vi "Re-Origin.vi"(1 "Transition":cluster{"X Delta":dbl, "Y Delta":dbl}, 2 "Coordinates":cluster{"X":dbl, "Y":dbl}[](array[cluster])) -> (0 "Normalized Coords":cluster{"X":dbl, "Y":dbl}[](array[cluster]))   [LabVIEW 2016]
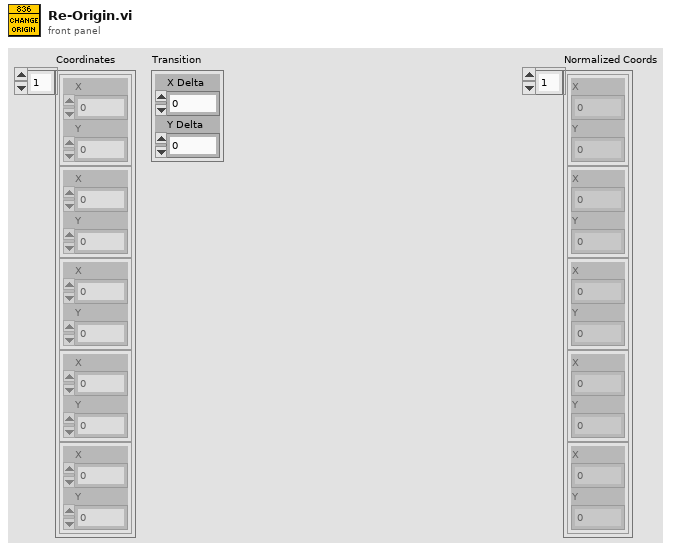
[diagram p1: front panel]
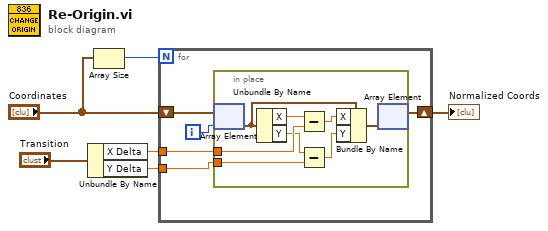
[diagram p0: block diagram]
diagram:
  n1 = Unbundle By Name("Transition") -> ("X Delta"=w3:dbl, "Y Delta"=w2:dbl)
  n2 = Array Size(array="Coordinates") -> (size(s)=w6:i32)
  n3 = for {
    N: w6 -> [_]
    tunnel: w3 -> [w9]
    tunnel: w2 -> [w8]
    shift-right: [w7] -> w1
    shift-left: "Coordinates" -> [w10]
    i -> [w11]
    n4 = in-place {
      in-place-border: w9 -> [w17]
      in-place-border: w8 -> [w15]
      n5 = in-place-array #1(w10, w11) -> (w18:cluster{"X":dbl, "Y":dbl})
      n6 = Unbundle By Name(w18) -> ("X"=w16:dbl, "Y"=w12:dbl)
      n7 = Subtract(x=w16, y=w17) -> (x-y=w14:dbl)
      n8 = Subtract(x=w12, y=w15) -> (x-y=w13:dbl)
      n9 = Bundle By Name(cluster=w18, "X"=w14, "Y"=w13) -> (w19:cluster{"X":dbl, "Y":dbl})
      n10 = in-place-array #1(w19) -> (w7:cluster{"X":dbl, "Y":dbl}[])  [unwired: 1 out]
    }
  }
  "Normalized Coords" <- w1
